vi "Calibrate-old.vi"   [LabVIEW 2018]
uses:
  Robot Global Data.vi
  <vilib>/Utility/file.llb/Write Delimited Spreadsheet (DBL).vi
types:
  T1 = typedef "WPI_AnalogChannelDevRef.ctl" = cluster{"DevStatus":errorcluster, "Analog Channel":T2}
  T2 = typedef "FPGA_AIChannel.ctl" = enum8{"AI 0", "AI 1", "AI 2", "AI 3", "AI MXP 0", "AI MXP 1", "AI MXP 2", "AI MXP 3", "Invalid"}
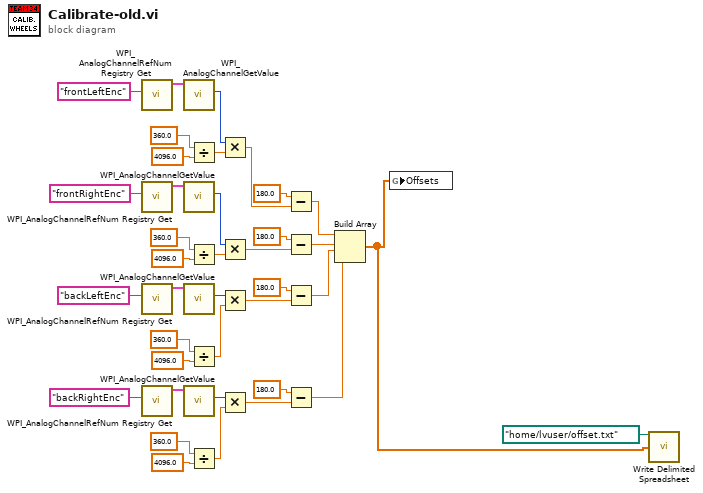
[diagram p0: block diagram]
diagram:
  n1 = call <vilib>:"WPI_AnalogChannelRefNum Registry Get.vi"("refnum name"="frontLeftEnc") -> ("AIDeviceRef"=w19:T1)  [unwired: 9 in, 1 out]
  n2 = call <vilib>:"WPI_AnalogChannelRefNum Registry Get.vi"("refnum name"="frontRightEnc") -> ("AIDeviceRef"=w22:T1)  [unwired: 9 in, 1 out]
  n3 = call <vilib>:"WPI_AnalogChannelRefNum Registry Get.vi"("refnum name"="backLeftEnc") -> ("AIDeviceRef"=w31:T1)  [unwired: 9 in, 1 out]
  n4 = call <vilib>:"WPI_AnalogChannelRefNum Registry Get.vi"("refnum name"="backRightEnc") -> ("AIDeviceRef"=w34:T1)  [unwired: 9 in, 1 out]
  n5 = call <vilib>:"WPI_AnalogChannelGetValue.vi"("AIDeviceRef"=w19) -> ("Value"=w20:i16)  [unwired: 8 in, 2 out]
  n6 = call <vilib>:"WPI_AnalogChannelGetValue.vi"("AIDeviceRef"=w22) -> ("Value"=w21:i16)  [unwired: 8 in, 2 out]
  n7 = call <vilib>:"WPI_AnalogChannelGetValue.vi"("AIDeviceRef"=w31) -> ("Value"=w32:i16)  [unwired: 8 in, 2 out]
  n8 = call <vilib>:"WPI_AnalogChannelGetValue.vi"("AIDeviceRef"=w34) -> ("Value"=w33:i16)  [unwired: 8 in, 2 out]
  n9 = Divide(x=360.0, y=4096.0) -> (x/y=w16:dbl)
  n10 = Divide(x=360.0, y=4096.0) -> (x/y=w25:dbl)
  n11 = Divide(x=360.0, y=4096.0) -> (x/y=w28:dbl)
  n12 = Divide(x=360.0, y=4096.0) -> (x/y=w37:dbl)
  n13 = Multiply(x=w20, y=w16) -> (x*y=w10:dbl)
  n14 = Multiply(x=w21, y=w25) -> (x*y=w9:dbl)
  n15 = Multiply(x=w32, y=w28) -> (x*y=w8:dbl)
  n16 = Multiply(x=w33, y=w37) -> (x*y=w7:dbl)
  n17 = Subtract(x=180.0 ("y"), y=w10) -> (x-y=w5:dbl)
  n18 = Subtract(x=180.0 ("y"), y=w9) -> (x-y=w4:dbl)
  n19 = Subtract(x=180.0 ("y"), y=w8) -> (x-y=w3:dbl)
  n20 = Subtract(x=180.0 ("y"), y=w7) -> (x-y=w2:dbl)
  n21 = Build Array(w5, w4, w3, w2) -> (w1:dbl[])
  n22 = global write "Robot Global Data.vi" "Offsets"(w1) -> ()
  n23 = call-poly <vilib>:"Write Delimited Spreadsheet.vi"("file path (dialog if empty)"=path "/home/lvuser/offset.txt", "1D data"=w1) -> ()  [unwired: 12 in, 2 out]
